vi "Strict enable disable.vi"(9 "Disabled":T1(array[ring]), 11 "Ref in":refnum<vi>[](array[refnum])) -> ()   [LabVIEW 2020]
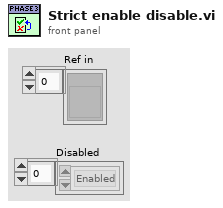
[diagram p1: front panel]
types:
  T1 = enum8{"Enabled", "Disabled", "Disabled and Grayed Out"}[]
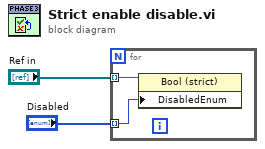
[diagram p0: block diagram]
diagram:
  n1 = for {
    tunnel: "Disabled" -> [w3] mode=indexing
    tunnel: "Ref in" -> [w4] mode=indexing
    n2 = property on="Property Node" class="Bool (strict)"(reference=w4, "DisabledEnum"=w3) -> ()  [unwired: 1 in, 2 out]
  }
